vi "Camera.vi"() -> ()   [LabVIEW 2013]
uses:
  <vilib>/Utility/miscctls.llb/LVPoint32TypeDef.ctl
  <vilib>/vision/driver/NI_Vision_Acquisition_Software.lvlib
panel:
  in  "ShutDownSystem":bool
  out "Coords":T1
  out "Image":T2(plugin-control)
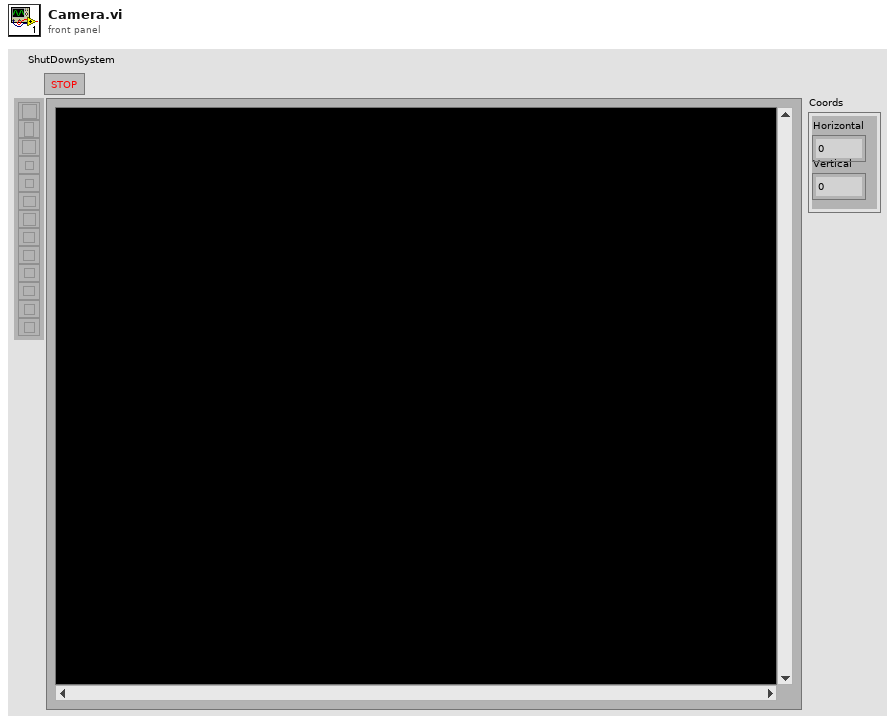
[diagram p1: front panel]
types:
  T1 = typedef "LVPoint32TypeDef.ctl" = cluster{"Horizontal":i32, "Vertical":i32}
  T2 = typedef "IMAQ Image.ctl" = refnum<image>
  T3 = cluster{"Type":u32, "Version":u32, "Flags":u32, "SerialNumberHigh":u32, "SerialNumberLow":u32, "BusType":u32, "InterfaceName":string, "VendorName":string, "ModelName":string, "CameraFileName":string, "CameraAttributeURL":string}[]
  T4 = cluster{"Type":u32, "Version":u32, "Flags":u32, "SerialNumberHigh":u32, "SerialNumberLow":u32, "BusType":u32, "InterfaceName":string, "VendorName":string, "ModelName":string, "CameraFileName":string, "CameraAttributeURL":string}
  T5 = typedef "IMAQdx.ctl" = refnum<k21>
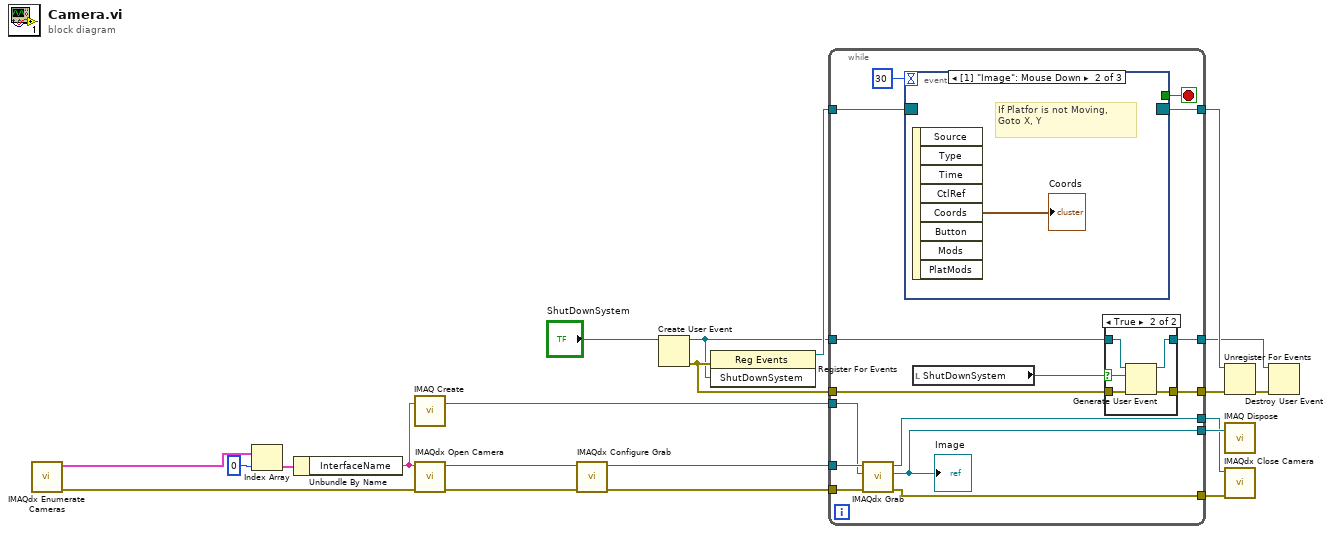
[diagram p0: block diagram]
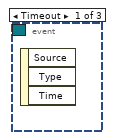
[diagram p3: hidden frame]
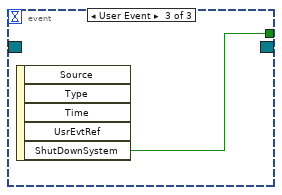
[diagram p4: hidden frame]
diagram:
  n1 = call <vilib>:"IMAQdx Enumerate Cameras.vi"() -> ("error out"=w11:errorcluster, "Camera Information Array"=w8:T3)  [unwired: 10 in]
  n2 = Index Array(array=w8, index=0) -> (element=w10:T4)
  n3 = Unbundle By Name(w10) -> ("InterfaceName"=w19:string)
  n4 = call "IMAQ Create"("Image Name"=w19) -> ("New Image"=w13:T2)  [unwired: 4 in, 1 out]
  n5 = call <vilib>:"IMAQdx Open Camera.vi"("error in"=w11, "Session In"=w19) -> ("error out"=w18:errorcluster, "Session Out"=w20:T5)  [unwired: 8 in]
  n6 = call <vilib>:"IMAQdx Configure Grab.vi"("error in"=w18, "Session In"=w20) -> ("error out"=w17:errorcluster, "Session Out"=w12:T5)  [unwired: 8 in]
  n7 = Create User Event(user event datatype="ShutDownSystem") -> (user event=w3:refnum<user-event>, error out=w4:errorcluster)  [unwired: 1 in]
  n8 = register-events(error in=w4, w3) -> (reference out=w6:refnum<event-registration>)  [unwired: 1 in, 1 out]
  n9 = while {
    tunnel: w17 -> [w36]
    tunnel: w12 -> [w35]
    tunnel: w13 -> [w34]
    tunnel: [w33] -> w14
    tunnel: [w32] -> w15
    tunnel: [w31] -> w16
    tunnel: [w29] -> w7
    tunnel: w6 -> [w28]
    tunnel: w4 -> [w27]
    tunnel: w3 -> [w26]
    tunnel: [w25] -> w2
    tunnel: [w23] -> w1
    stop <- w24 stop-if-true
    n10 = call <vilib>:"IMAQdx Grab.vi"("error in"=w36, "Image In"=w34, "Session In"=w35) -> ("error out"=w33:errorcluster, "Image Out"=w31:T2, "Session Out"=w32:T5)  [unwired: 5 in, 1 out]
    "Image" <- w31
    n11 = event shown="[1] \"Image\": Mouse Down" {
      selector: w28 -> [_ _ _]
      dyn-events: [_ _ _] -> w29
      timeout: 30 -> [_ _ _]
      tunnel: [_ _ w45] -> w24
      event Timeout {
        n12 = event-data() -> ()  [unwired: 1 in, 3 out]
      }
      event "Image": Mouse Down {
        # "If Platfor is not Moving,\nGoto X, Y"
        n13 = event-data() -> ("Coords"=→"Coords":T1)  [unwired: 1 in, 7 out]
      }
      event User Event {
        n14 = event-data() -> ("ShutDownSystem"=w45:bool)  [unwired: 1 in, 4 out]
      }
    }
    n15 = local read "ShutDownSystem"() -> (w22:bool)
    n16 = case shown="True" w22 {
      selector: w22 -> [_ w43]
      tunnel: w27 -> [w38 w41]
      tunnel: [w38 w42] -> w25
      tunnel: w26 -> [w37 w40]
      tunnel: [w37 w39] -> w23
      frame False {
      }
      frame True {
        n17 = Generate User Event(user event=w40, event data cluster=w43, error in=w41) -> (user event out=w39:refnum<user-event>, error out=w42:errorcluster)  [unwired: 1 in]
      }
    }
  }
  n18 = Unregister For Events(event registration refnum=w7, error in=w2) -> (error out=w21:errorcluster)
  n19 = call "IMAQ Dispose"("Image"=w16) -> ()  [unwired: 5 in, 1 out]
  n20 = call <vilib>:"IMAQdx Close Camera.vi"("error in"=w14, "Session In"=w15) -> ()  [unwired: 9 in, 1 out]
  n21 = Destroy User Event(user event=w1, error in=w21) -> ()  [unwired: 1 out]
